vi "SW_Draw_mouse.vi"(0 "Input picture (background)":picture, 5 "Pixels per mm":dbl, 7 "Mouse coord X, mm":dbl, 9 "Mouse coord Y, mm":dbl, 11 "Mouse angle of rotation, deg":dbl) -> (4 "Output picture (with mouse overlay)":picture)   [LabVIEW 2016]
panel:
  in  "Mouse initial picture height, pix":u16
  in  "Mouse initial picture width, pix":u16
  in  "Mouse color":u32(colorbox)
  in  "Mouse size, mm":dbl
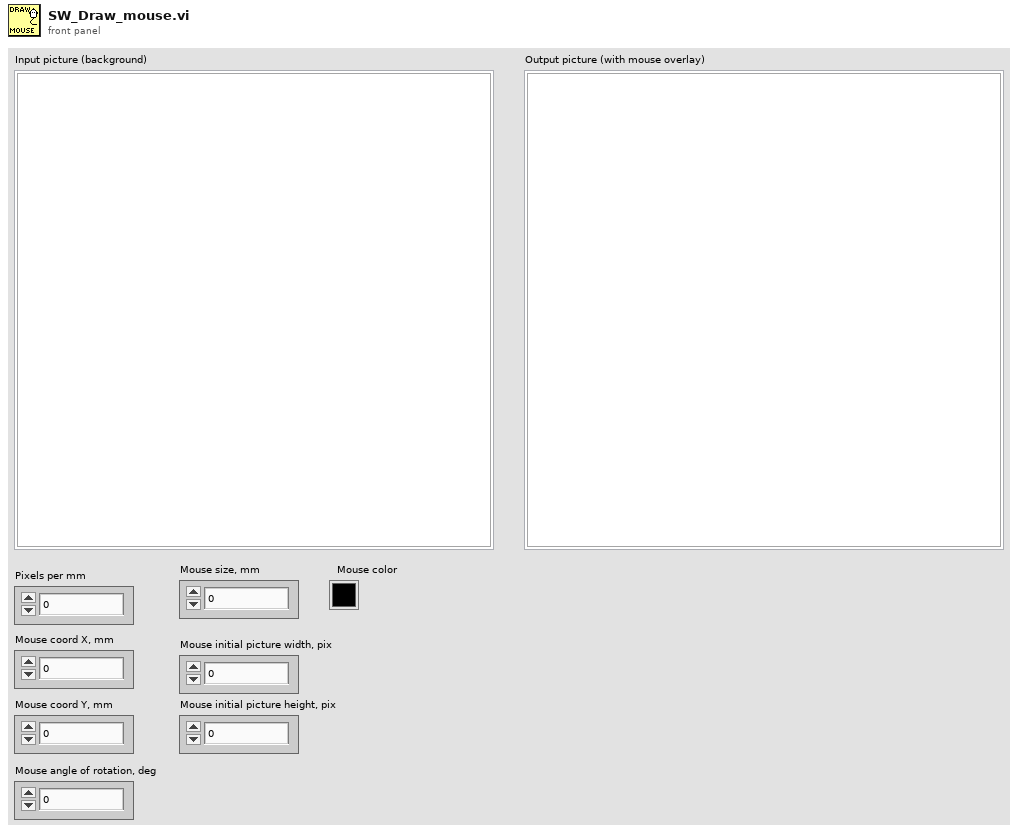
[diagram p1: front panel]
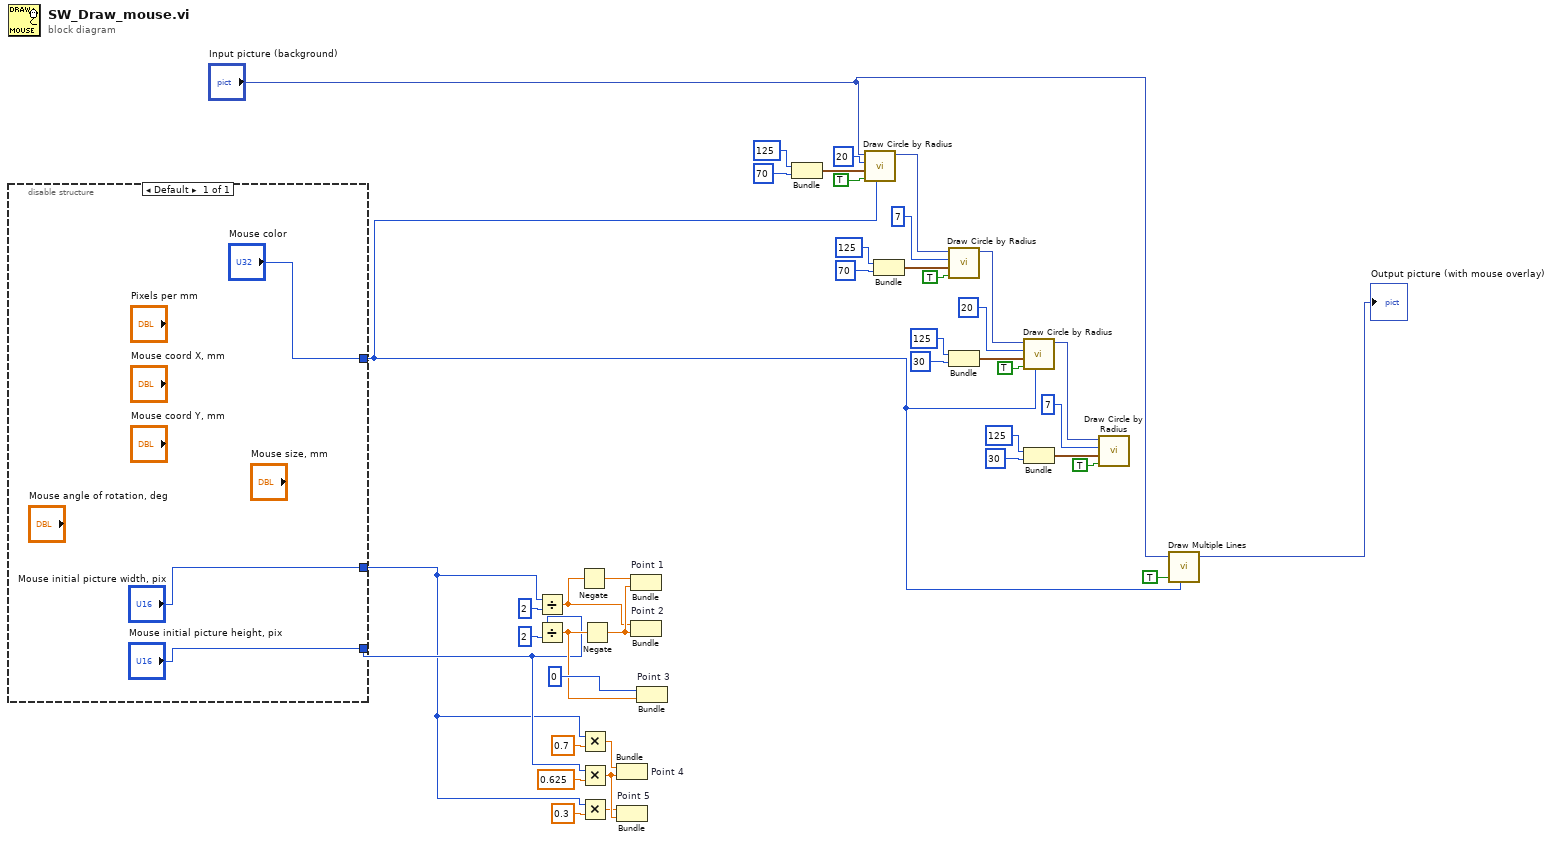
[diagram p0: block diagram]
diagram:
  n1 = disable-structure shown="Default" {
    disable-tunnel: ["Mouse color"] -> w30
    disable-tunnel: ["Mouse initial picture width, pix"] -> w2
    disable-tunnel: ["Mouse initial picture height, pix"] -> w5
    frame Enabled {
    }
  }
  n2 = Divide(x=w2, y=u16 2) -> (x/y=w12:dbl)
  n3 = Divide(x=w5, y=u16 2) -> (x/y=w10:dbl)
  n4 = Negate(x=w12) -> (-x=w14:dbl)
  n5 = Multiply(x=w2, y=0.7) -> (x*y=w7:dbl)
  n6 = Multiply(x=w5, y=0.625) -> (x*y=w4:dbl)
  n7 = Multiply(x=w2, y=0.3) -> (x*y=w1:dbl)
  n8 = Negate(x=w10) -> (-x=w13:dbl)
  n9 = Bundle "Point 4"(w7, w4) -> ()  [unwired: 1 in, 1 out]
  n10 = Bundle "Point 5"(w1, w4) -> ()  [unwired: 1 in, 1 out]
  n11 = Bundle "Point 1"(w14, w13) -> ()  [unwired: 1 in, 1 out]
  n12 = Bundle "Point 2"(w12, w13) -> ()  [unwired: 1 in, 1 out]
  n13 = Bundle "Point 3"(0, w10) -> ()  [unwired: 1 in, 1 out]
  n14 = Bundle(125, 70) -> (w39:cluster{i32, i32})  [unwired: 1 in]
  n15 = call <vilib>:"Draw Circle by Radius.vi"("color(black)"=w30, "fill?(F)"=TRUE, "pixel center"=w39, "radius"=i16 20, "picture"="Input picture (background)") -> ("new picture"=w24:picture)  [unwired: 6 in]
  n16 = Bundle(125, 70) -> (w27:cluster{i32, i32})  [unwired: 1 in]
  n17 = call <vilib>:"Draw Circle by Radius.vi"("fill?(F)"=TRUE, "pixel center"=w27, "radius"=i16 7, "picture"=w24) -> ("new picture"=w23:picture)  [unwired: 7 in]
  n18 = Bundle(125, 30) -> (w33:cluster{i32, i32})  [unwired: 1 in]
  n19 = call <vilib>:"Draw Circle by Radius.vi"("color(black)"=w30, "fill?(F)"=TRUE, "pixel center"=w33, "radius"=i16 20, "picture"=w23) -> ("new picture"=w17:picture)  [unwired: 6 in]
  n20 = Bundle(125, 30) -> (w20:cluster{i32, i32})  [unwired: 1 in]
  n21 = call <vilib>:"Draw Circle by Radius.vi"("fill?(F)"=TRUE, "pixel center"=w20, "radius"=i16 7, "picture"=w17) -> ()  [unwired: 7 in, 1 out]
  n22 = call <vilib>:"Draw Multiple Lines.vi"("picture"="Input picture (background)", "fill?(F)"=TRUE, "color(black)"=w30) -> ("new picture"=→"Output picture (with mouse overlay)":picture)  [unwired: 6 in]
